vi "init.vi"(8 "error in":errorcluster, 11 "Analog_Input (in)":refnum<class "Analog_Input.lvclass">) -> (0 "error out":errorcluster, 3 "Analog_Input":refnum<class "Analog_Input.lvclass">)   [LabVIEW 2013, in "Analog_Input.lvclass"]
uses:
  Analog_Input.lvclass
  Analog_Input.lvclass/Analog_Input.ctl
  Globals.vi
  <vilib>/DAQmx/create/channels.llb/DAQmx Create Channel (AI-Voltage-Basic).vi
  <vilib>/DAQmx/configure/timing.llb/DAQmx Timing (Sample Clock).vi
  <vilib>/DAQmx/configure/trigger.llb/DAQmx Start Trigger (Digital Edge).vi
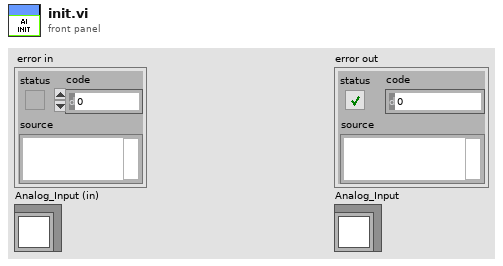
[diagram p1: front panel]
types:
  T1 = cluster{"Wait for start trigger?":bool, "source":tag, "edge":i32}
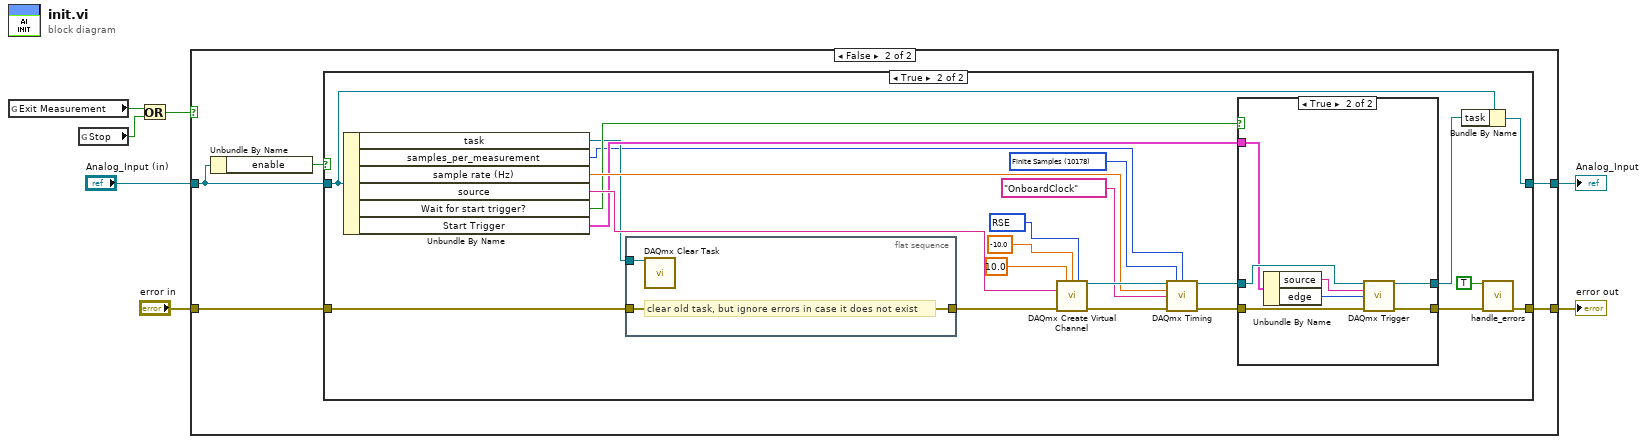
[diagram p0: block diagram]
diagram:
  n1 = global read "Globals.vi" "Exit Measurement"() -> (w3:bool)
  n2 = global read "Globals.vi" "Stop"() -> (w2:bool)
  n3 = Or(x=w3, y=w2) -> (x .or. y?=w1:bool)
  n4 = case shown="False" w1 {
    tunnel: "error in" -> [w9 w14]
    tunnel: [w9 w13] -> w6
    tunnel: "Analog_Input (in)" -> [w8 w11]
    tunnel: [w8 w12] -> w4
    frame True {
    }
    frame False {
      n5 = Unbundle By Name(w11) -> ("enable"=w10:bool)
      n6 = case shown="True" w10 {
        tunnel: w14 -> [w16 w19]
        tunnel: [w16 w32] -> w13
        tunnel: w11 -> [w15 w30]
        tunnel: [w15 w31] -> w12
        frame False {
        }
        frame True {
          w36 = 10178 items=["Finite Samples"=10178, "Continuous Samples"=10123, "Hardware Timed Single Point"=12522] ("sample mode")
          w39 = 10083 items=["default"=-1, "RSE"=10083, "NRSE"=10078, "Differential"=10106, "Pseudodifferential"=12529] ("input terminal configuration")
          n7 = Unbundle By Name(w30) -> ("task"=w20:refnum<k21>, "samples_per_measurement"=w17:i32, "sample rate (Hz)"=w29:dbl, "source"=w28:tag, "Wait for start trigger?"=w22:bool, "Start Trigger"=w21:T1)
          n8 = flat-sequence {
            tunnel: w19 -> [w40]
            tunnel: [w40] -> w18
            tunnel: w20 -> [w41]
            frame #0 {
              # "clear old task, but ignore errors in case it does not exist"
              n9 = call <vilib>:"DAQmx Clear Task.vi"("task in"=w41) -> ()  [unwired: 14 in, 1 out]
            }
          }
          n10 = call-poly <vilib>:"DAQmx Create Virtual Channel.vi"("maximum value"=10.0, "minimum value"=-10.0, "input terminal configuration"=w39, "physical channels"=w28, "error in"=w18) -> ("task out"=w38:refnum<k21>, "error out"=w37:errorcluster)  [unwired: 9 in]
          n11 = call-poly <vilib>:"DAQmx Timing.vi"("task/channels in"=w38, "sample mode"=w36, "samples per channel"=w17, "rate"=w29, "source"=tag "OnboardClock", "error in"=w37) -> ("task out"=w24:refnum<k21>, "error out"=w25:errorcluster)  [unwired: 8 in]
          n12 = case shown="True" w22 {
            tunnel: w24 -> [w43 w50]
            tunnel: [w43 w49] -> w23
            tunnel: w25 -> [w42 w48]
            tunnel: w21 -> [_ w47]
            tunnel: [w42 w44] -> w26
            frame False {
            }
            frame True {
              n13 = Unbundle By Name(w47) -> ("source"=w46:tag, "edge"=w45:i32)
              n14 = call-poly <vilib>:"DAQmx Trigger.vi"("task/channels in"=w50, "source"=w46, "edge"=w45, "error in"=w48) -> ("task out"=w49:refnum<k21>, "error out"=w44:errorcluster)  [unwired: 10 in]
            }
          }
          n15 = Bundle By Name(cluster=w30, "task"=w23) -> (w31:refnum<class "Analog_Input.lvclass">)
          n16 = call "handle_errors.vi"("Exit Operation"=TRUE, "error in (no error)"=w26) -> ("error out"=w32:errorcluster)  [unwired: 13 in]
        }
      }
    }
  }
  "error out" <- w6
  "Analog_Input" <- w4
